vi "Read degreesArc.vi"(8 "error in (no error)":errorcluster, 11 "Azimuth in":refnum<class "Azimuth.lvclass">) -> (0 "error out":errorcluster, 2 "degreesArc":dbl[unit] min=0.0 max=360.0, 3 "Azimuth out":refnum<class "Azimuth.lvclass">)   [LabVIEW 2014, in "TCSDataDefinitions.lvlib" / "TCSCommand.lvlib" / "TargetConfiguration.lvlib" / "Target.lvlib" / "FixedTarget.lvlib" / "Azimuth.lvclass"]
uses:
  Azimuth.lvclass
  Azimuth.lvclass/Azimuth.ctl
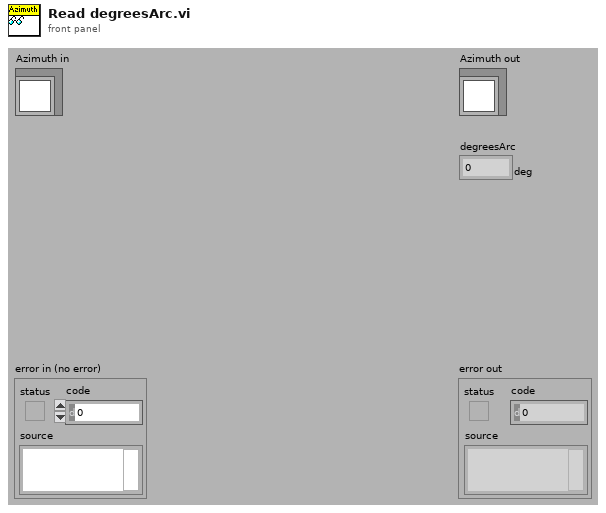
[diagram p1: front panel]
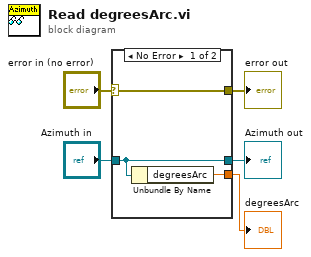
[diagram p0: block diagram]
diagram:
  n1 = case shown="No Error" "error in (no error)" {
    selector: "error in (no error)" -> [w8 w9]
    tunnel: [w8 w9] -> w4
    tunnel: [w7 w10] -> w2
    tunnel: "Azimuth in" -> [w7 w10]
    tunnel: [w6 _] -> w1
    frame No Error {
      n2 = Unbundle By Name(w7) -> ("degreesArc"=w6:dbl[unit])
    }
    frame Error {
    }
  }
  "error out" <- w4
  "Azimuth out" <- w2
  "degreesArc" <- w1
